vi "main_V2 _1.vi"() -> ()   [LabVIEW 2019]
doc: "This VI takes input from HMI (Nextion 7inch enhanced version) DIOs, emergency button (used as interlocking) and mode (Auto/manual) button from hardware. After getting inputs it will operate the Jacks either manual or in auto mode."
uses:
  <vilib>/myRIO/Instrument Drivers/Onboard IO/DIO/typedefs/DIO Reference.ctl
  <vilib>/myRIO/Common/Instrument Driver Framework/Utilities/typedefs/myRIO Generic Hardware Reference.ctl
  <vilib>/myRIO/Common/Instrument Driver Framework/Utilities/typedefs/Hardware Version Enum.ctl
  <vilib>/myRIO/Common/Instrument Driver Framework/Utilities/typedefs/myRIO v1.0 Reference.ctl
  <vilib>/myRIO/Common/Instrument Driver Framework/Utilities/typedefs/Generic FPGA Reference.ctl
  <vilib>/myRIO/Common/Instrument Driver Framework/myRIO v1.0/DIO/typedefs/DIO Channels List.ctl
  <vilib>/myRIO/Common/Instrument Driver Framework/myRIO v1.0/DIO/typedefs/DIO Channels Enum.ctl
  <vilib>/userDefined/High Color/nirio_resource_hc.ctl
  <vilib>/myRIO/Common/Instrument Driver Framework/Utilities/vis/Is FPGA Ref Available.vi
  <vilib>/myRIO/Common/Instrument Driver Framework/myRIO v1.0/DIO/vis/myRIO v1.1 Open DIO.vi
  <vilib>/myRIO/Instrument Drivers/Onboard IO/DIO/vis/Read.vi
  <vilib>/myRIO/Instrument Drivers/Onboard IO/DIO/vis/Write.vi
  <vilib>/myRIO/Common/Instrument Driver Framework/Utilities/vis/Validate Channels.vi
  <vilib>/myRIO/Common/Instrument Driver Framework/myRIO v1.0/DIO/vis/myRIO v1.0 Reserve DIO.vi
  <vilib>/myRIO/Common/Instrument Driver Framework/myRIO v1.0/Resource Manager/vis/myRIO v1.0 Reserve Channel List.vi
  <vilib>/myRIO/Common/Instrument Driver Framework/myRIO v1.0/DIO/vis/myRIO v1.0 Build MUX Configuration DIO.vi
  <vilib>/myRIO/Common/Instrument Driver Framework/myRIO v1.0/Resource Manager/vis/myRIO v1.0 Reserve Channel.vi
  <vilib>/myRIO/Common/Instrument Driver Framework/myRIO v1.0/Resource Manager/vis/myRIO v1.0 Unreserve Channel.vi
  <vilib>/myRIO/Common/Instrument Driver Framework/myRIO v1.0/Resource Manager/vis/myRIO v1.0 Create Configuration List.vi
  <vilib>/myRIO/Common/Instrument Driver Framework/myRIO v1.0/Resource Manager/vis/myRIO v1.0 Build Mutex Name.vi
  <vilib>/Utility/VariantDataType/GetNumericInfo.vi
  <vilib>/Utility/error.llb/Error Cluster From Error Code.vi
  <vilib>/myRIO/Common/Instrument Driver Framework/myRIO v1.0/myRIO v1.1 Open.vi
  <vilib>/myRIO/Common/Instrument Driver Framework/Utilities/vis/IO Manager.vi
  <vilib>/myRIO/Common/Instrument Driver Framework/Utilities/vis/Configuration Manager.vi
  <vilib>/myRIO/Common/Instrument Driver Framework/myRIO v1.0/Resource Manager/vis/myRIO v1.0 Configure IO.vi
  <vilib>/myRIO/Common/Instrument Driver Framework/myRIO v1.0/myRIO v1.0 Close.vi
  <vilib>/myRIO/Common/Instrument Driver Framework/myRIO v1.0/DIO/vis/myRIO v1.0 Read DIO.vi
  <vilib>/myRIO/Common/Instrument Driver Framework/myRIO v1.0/DIO/vis/myRIO v1.0 Write DIO.vi
  <vilib>/myRIO/Express VI/Onboard IO/DI/DI Express VI.xnode
  <vilib>/myRIO/Instrument Drivers/Onboard IO/DIO/vis/myRIO DIO Open.xnode
  <vilib>/myRIO/Express VI/Onboard IO/DO/DO Express VI.xnode
  <vilib>/myRIO/Instrument Drivers/Onboard IO/DIO/DIO.lvlib
panel:
  out "timerst":i32
  in  "Reset":bool
  out "Elapsed Time (s)":dbl format="%#_2g"
  out "levell check":i32
  out "1":bool
  out "X Axis":dbl
  out "Y Axis":dbl
  out "8":bool
  out "7":bool
  out "4":bool
  out "3":bool
  out "6":bool
  out "5":bool
  out "2":bool
  out "Numeric":i32
  out "Numeric 2":i32
  out "AutoLevel":bool
  out "WithDrawAll":bool
  out "Emergency stop":bool
  out "z":i16
  out "Temp":dbl
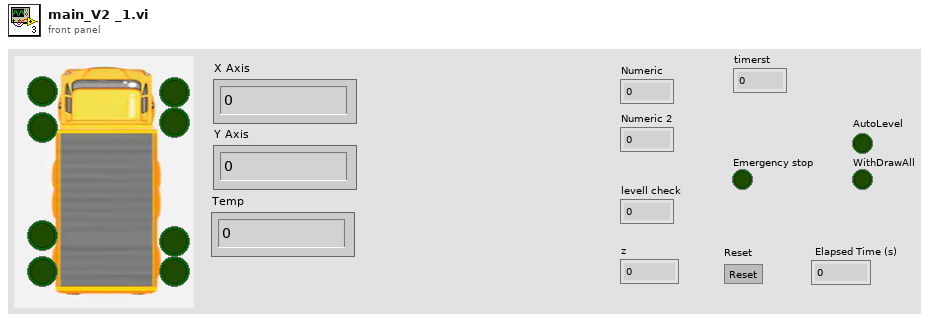
[diagram p1: front panel]
types:
  T1 = typedef "DIO.lvlib/DIO Reference.ctl" = cluster{"myRIO Reference":T2, "DIO Channels List":T6}
  T2 = typedef "myRIO Generic Hardware Reference.ctl" = cluster{"myRIO Model":T3, "myRIO Hardware Reference":T4}
  T3 = typedef "Hardware Version Enum.ctl" = enum16{"Unknown", "myRIO-1900", "myRIO-1950", "roboRIO", "NI ELVIS RIO CM", "ELVIS III"}
  T4 = typedef "myRIO v1.0 Reference.ctl" = cluster{"Generic FPGA Reference":T5, "Allow multiple opens":bool}
  T5 = typedef "Generic FPGA Reference.ctl" = refnum<k20>
  T6 = typedef "DIO Channels List.ctl" = T7[]
  T7 = typedef "DIO Channels Enum.ctl" = enum16{"Not Connected", "C/DIO0", "C/DIO1", "C/DIO2", "C/DIO3", "C/DIO4", "C/DIO5", "C/DIO6", "C/DIO7", "A/DIO0", "A/DIO1", "A/DIO2", "A/DIO3", "A/DIO4", "A/DIO5", "A/DIO6", "A/DIO7", "A/DIO8", "A/DIO9", "A/DIO10", "A/DIO11", "A/DIO12", "A/DIO13", "A/DIO14", "A/DIO15", "A/DIO16", "A/DIO17", "A/DIO18", "A/DIO19", "B/DIO0", "B/DIO1", "B/DIO2", "B/DIO3", "B/DIO4", "B/DIO5", "B/DIO6", "B/DIO7", "B/DIO8", "B/DIO9", "B/DIO10", "B/DIO11", "B/DIO12", "B/DIO13", "B/DIO14", "B/DIO15", "B/DIO16", "B/DIO17", "B/DIO18", "B/DIO19", "LED0", "LED1", "LED2", "LED3", "Button0", "DIO/DIO0", "DIO/DIO1", "DIO/DIO2", "DIO/DIO3", "DIO/DIO4", "DIO/DIO5", "DIO/DIO6", "DIO/DIO7", "DIO/DIO8", "DIO/DIO9", "SPI/CS0", "SPI/CS1", "SPI/CS2", "SPI/CS3", "LED RADIO (Green)", "LED RADIO (Red)", "LED COMM (Green)", "LED COMM (Red)", "LED MODE (Green)", "LED MODE (Red)"}
  T8 = typedef "nirio_resource_hc.ctl" = tag
  T9 = cluster{"Boolean array[0]":bool, "Boolean array[1]":bool, "Boolean array[2]":bool, "Boolean array[3]":bool, "Boolean array[4]":bool, "Boolean array[5]":bool, "Boolean array[6]":bool, "Boolean array[7]":bool}
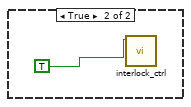
[diagram p3: hidden frame]
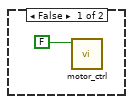
[diagram p6: hidden frame]
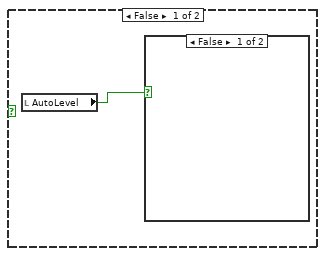
[diagram p7: hidden frame]
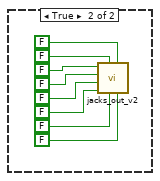
[diagram p8: hidden frame]
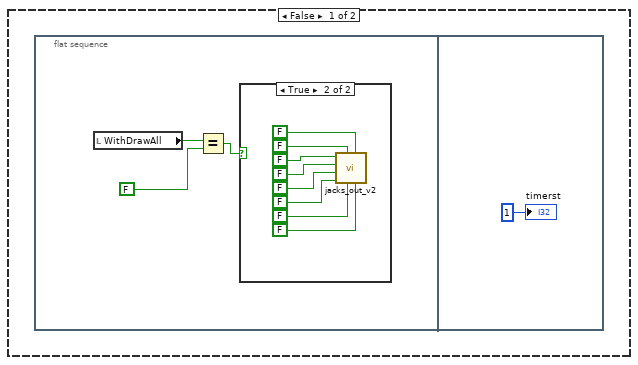
[diagram p9: hidden frame]
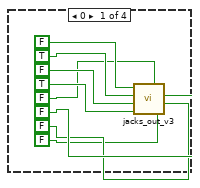
[diagram p11: hidden frame]
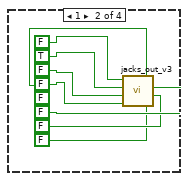
[diagram p12: hidden frame]
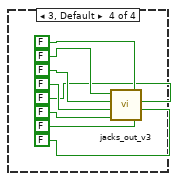
[diagram p13: hidden frame]
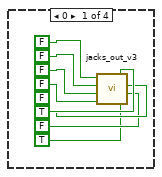
[diagram p14: hidden frame]
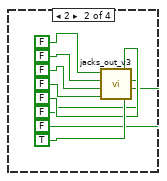
[diagram p15: hidden frame]
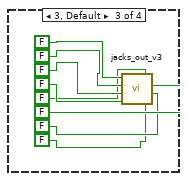
[diagram p16: hidden frame]
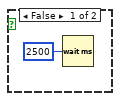
[diagram p19: hidden frame]
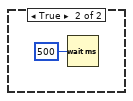
[diagram p20: hidden frame]
diagram:
  n1 = while {
    shift-right: [w16] -> _
    shift-left: 0 -> [w17]
    shift-right: [w7] -> _
    shift-left: 0 -> [w9]
    i -> [w15]
    stop <- FALSE ("stop") stop-if-true
    n2 = flat-sequence {
      tunnel: w17 -> [w21]
      tunnel: [w21] -> w14
      tunnel: [w19] -> w11
      tunnel: [w20] -> w10
      tunnel: w9 -> [w20]
      tunnel: w14 -> [w61]
      tunnel: [w60] -> w6
      tunnel: w11 -> [w59]
      tunnel: w10 -> [w58]
      tunnel: [w57] -> w5
      tunnel: w6 -> [w823]
      tunnel: [w823] -> w13
      tunnel: [w819] -> w8
      tunnel: w5 -> [w819]
      tunnel: w13 -> [w835]
      tunnel: w8 -> [w831]
      tunnel: [w835] -> w4
      tunnel: [w831] -> w3
      tunnel: [w849] -> w7
      tunnel: [w850] -> w16
      tunnel: w4 -> [w850]
      tunnel: w3 -> [w849]
      frame #0 {
        # "True for Manual and False for Auto"
        n3 = xnode "Button_inputs"() -> ("MANUAL/SFTWRE (A/DIO9 (Pin 29))"=w18:bool)  [unwired: 1 in, 1 out]
        n4 = Not(x=w18) -> (.not. x?=w19:bool)
        "Emergency stop" <- w19
      }
      frame #1 {
        # "Emergency stop case"
        n5 = case shown="True" w59 {
          tunnel: w61 -> [_ w148]
          tunnel: [0 w150] -> w60
          tunnel: w58 -> [_ w146]
          tunnel: [0 w145] -> w57
          frame False {
            n6 = flat-sequence {
              frame #0 {
                n7 = xnode "Digital output (1 sample) 4"("contactor (A/DIO3 (Pin 17))"=FALSE) -> ()  [unwired: 1 in, 1 out]
              }
              frame #1 {
                n8 = xnode "Interlock"("interlock_relay (A/DIO4 (Pin 19))"=FALSE ("interlock_relay (B/DIO8 (Pin 27))")) -> ()  [unwired: 1 in, 1 out]
              }
              frame #2 {
                n9 = call "jacks_out_v2.vi"("J4dn"=FALSE ("R6 (B/DIO13 (Pin 26))"), "J1up"=FALSE ("R3 (B/DIO2 (Pin 15))"), "J4up"=FALSE ("R5 (B/DIO4 (Pin 19))"), "J1dn"=FALSE ("R2 (B/DIO1 (Pin 13))"), "J3dn"=FALSE ("R4 (B/DIO3 (Pin 17))"), "J3up"=FALSE ("R7 (B/DIO14 (Pin 32))"), "J2dn"=FALSE ("R8 (B/DIO15 (Pin 34))"), "J2up"=FALSE ("R1 (B/DIO0 (Pin 11))")) -> ()  [unwired: 4 in]
              }
              frame #3 {
                n10 = local write "levell check"(0 ("levell check")) -> ()
              }
            }
          }
          frame True {
            n11 = flat-sequence {
              tunnel: [w154] -> w149
              tunnel: w148 -> [w154]
              tunnel: [w152] -> w147
              tunnel: w146 -> [w152]
              tunnel: [w161] -> w150
              tunnel: w149 -> [w160]
              tunnel: w147 -> [w159]
              tunnel: [w158] -> w145
              frame #0 {
                n12 = call "interlock_ctrl.vi"("Interlock"=TRUE ("interlock_relay (B/DIO8 (Pin 27))")) -> ()  [unwired: 7 in]
                n13 = Wait (ms)(milliseconds to wait=u32 50) -> ()  [unwired: 1 out]
              }
              frame #1 {
                # "Manual/Auto case"
                n14 = call "Nextion_PageRead.vi"() -> ("pageNo"=w157:u8)  [unwired: 10 in, 1 out]
                n15 = Equal?(x=w157, y=u8 1) -> (x = y?=w155:bool)
                n16 = case "Auto/Manual Case" shown="False" w155 {
                  tunnel: [w164 0] -> w161
                  tunnel: w160 -> [w162 _]
                  tunnel: w159 -> [_ w507]
                  tunnel: [0 w506] -> w158
                  frame False {
                    # "cccvv"
                    n17 = flat-sequence {
                      tunnel: w162 -> [w167]
                      frame #0 {
                        n18 = Equal?(x=w167, y=0) -> (x = y?=w165:bool)
                        n19 = case shown="True" w165 {
                          frame False {
                          }
                          frame True {
                            n20 = Wait (ms)(milliseconds to wait=u32 100) -> ()  [unwired: 1 out]
                            n21 = call "Nextion_Write.vi"("string"="page page0") -> ()  [unwired: 10 in, 1 out]
                            n22 = call "jacks_out_v3.vi"("J4 DOWN"=FALSE ("R6 (B/DIO13 (Pin 26))"), "J4 UP"=FALSE ("R5 (B/DIO4 (Pin 19))"), "J3 DOWN"=FALSE ("R4 (B/DIO3 (Pin 17))"), "J3 UP"=FALSE ("R7 (B/DIO14 (Pin 32))"), "J2 DOWN"=FALSE ("R8 (B/DIO15 (Pin 34))"), "J2 UP"=FALSE ("R1 (B/DIO0 (Pin 11))"), "J1 DOWN"=FALSE ("R2 (B/DIO1 (Pin 13))"), "J1 UP"=FALSE ("R3 (B/DIO2 (Pin 15))")) -> ()
                            "levell check" <- 0
                          }
                        }
                      }
                      frame #1 {
                        n23 = flat-sequence {
                          frame #0 {
                            n24 = call "Nextion_buttonRead.vi"("string"="get bt0.val") -> ("Bt_val"=w187:u8, "ref"=w186:u8)  [unwired: 8 in, 1 out]
                            n25 = Wait (ms)(milliseconds to wait=u32 50) -> ()  [unwired: 1 out]
                            n26 = Equal?(x=w187, y=u8 1) -> (x = y?=w185:bool)
                            n27 = Equal?(x=u8 113, y=w186) -> (x = y?=w184:bool)
                            n28 = And(x=w184, y=w185) -> (x .and. y?=→"AutoLevel":bool)
                          }
                          frame #1 {
                            n29 = call "Nextion_buttonRead.vi"("string"="get bt1.val") -> ("Bt_val"=w190:u8, "ref"=w191:u8)  [unwired: 8 in, 1 out]
                            n30 = Wait (ms)(milliseconds to wait=u32 50) -> ()  [unwired: 1 out]
                            n31 = Equal?(x=u8 113, y=w191) -> (x = y?=w193:bool)
                            n32 = Equal?(x=w190, y=u8 1) -> (x = y?=w192:bool)
                            n33 = And(x=w193, y=w192) -> (x .and. y?=→"WithDrawAll":bool)
                          }
                          frame #2 {
                            n34 = local read "WithDrawAll"() -> (w198:bool)
                            n35 = local read "AutoLevel"() -> (w199:bool)
                            n36 = Or(x=w199, y=w198) -> (x .or. y?=w197:bool)
                            n37 = case shown="True" w197 {
                              frame False {
                                n38 = call "motor_ctrl.vi"("Motor"=FALSE ("contactor (A/DIO3 (Pin 17))")) -> ()  [unwired: 7 in]
                              }
                              frame True {
                                n39 = call "motor_ctrl.vi"("Motor"=TRUE ("contactor (A/DIO3 (Pin 17))")) -> ()  [unwired: 7 in]
                              }
                            }
                          }
                          frame #3 {
                            n40 = local read "WithDrawAll"() -> (w203:bool)
                            n41 = case shown="True" w203 {
                              frame False {
                                n42 = local read "AutoLevel"() -> (w204:bool)
                                n43 = case shown="False" w204 {
                                frame False {
                                }
                                frame True {
                                n44 = call "jacks_out_v2.vi"("J4dn"=FALSE ("R6 (B/DIO13 (Pin 26))"), "J1up"=FALSE ("R3 (B/DIO2 (Pin 15))"), "J4up"=FALSE ("R5 (B/DIO4 (Pin 19))"), "J1dn"=FALSE ("R2 (B/DIO1 (Pin 13))"), "J3dn"=FALSE ("R4 (B/DIO3 (Pin 17))"), "J3up"=FALSE ("R7 (B/DIO14 (Pin 32))"), "J2dn"=FALSE ("R8 (B/DIO15 (Pin 34))"), "J2up"=FALSE ("R1 (B/DIO0 (Pin 11))")) -> ()  [unwired: 4 in]
                                }
                                }
                              }
                              frame True {
                                n45 = local write "levell check"(0 ("levell check")) -> ()
                                n46 = call "jacks_out_v3.vi"("J4 DOWN"=FALSE ("R6 (B/DIO13 (Pin 26))"), "J4 UP"=TRUE ("R5 (B/DIO4 (Pin 19))"), "J3 DOWN"=FALSE ("R4 (B/DIO3 (Pin 17))"), "J3 UP"=TRUE ("R7 (B/DIO14 (Pin 32))"), "J2 DOWN"=FALSE ("R8 (B/DIO15 (Pin 34))"), "J2 UP"=TRUE ("R1 (B/DIO0 (Pin 11))"), "J1 DOWN"=FALSE ("R2 (B/DIO1 (Pin 13))"), "J1 UP"=TRUE ("R3 (B/DIO2 (Pin 15))")) -> ()
                              }
                            }
                            n47 = Wait (ms)(milliseconds to wait=u32 50) -> ()  [unwired: 1 out]
                          }
                          frame #4 {
                          }
                          frame #5 {
                            n48 = local read "AutoLevel"() -> (w222:bool)
                            n49 = case shown="True" w222 {
                              frame False {
                                n50 = flat-sequence {
                                frame #0 {
                                n51 = local read "WithDrawAll"() -> (w224:bool)
                                n52 = Equal?(x=w224, y=FALSE) -> (x = y?=w225:bool)
                                n53 = case shown="True" w225 {
                                frame False {
                                }
                                frame True {
                                n54 = call "jacks_out_v2.vi"("J4dn"=FALSE ("R6 (B/DIO13 (Pin 26))"), "J1up"=FALSE ("R3 (B/DIO2 (Pin 15))"), "J4up"=FALSE ("R5 (B/DIO4 (Pin 19))"), "J1dn"=FALSE ("R2 (B/DIO1 (Pin 13))"), "J3dn"=FALSE ("R4 (B/DIO3 (Pin 17))"), "J3up"=FALSE ("R7 (B/DIO14 (Pin 32))"), "J2dn"=FALSE ("R8 (B/DIO15 (Pin 34))"), "J2up"=FALSE ("R1 (B/DIO0 (Pin 11))")) -> ()  [unwired: 4 in]
                                }
                                }
                                }
                                frame #1 {
                                "timerst" <- 1
                                }
                                }
                              }
                              frame True {
                                n55 = flat-sequence {
                                frame #0 {
                                n56 = local read "timerst"() -> (w240:i32)
                                n57 = Equal?(x=w240, y=1) -> (x = y?=w235:bool)
                                n58 = Select(t=TRUE ("Reset"), s=w235, f=FALSE ("Reset")) -> (s? t:f=w238:bool)
                                n59 = local write "Reset"(w238) -> ()
                                }
                                frame #1 {
                                n60 = flat-sequence {
                                tunnel: [w242] -> w241
                                tunnel: w241 -> [w244]
                                frame #0 {
                                n61 = call "Elapsed Time"("Reset"="Reset") -> ("Elapsed Time (s)"=w242:dbl)  [unwired: 11 in, 7 out]
                                "Elapsed Time (s)" <- w242
                                }
                                frame #1 {
                                n62 = Multiply(x=w244, y=10.0) -> (x*y=w246:dbl)
                                n63 = To Word Integer(number=w246) -> (16bit integer=w245:i16)
                                n64 = Format Into String(initial string="x2.val=", w245) -> (resulting string=w248:string)  [unwired: 2 in, 1 out]
                                n65 = call "Nextion_Write.vi"("string"=w248) -> ()  [unwired: 10 in, 1 out]
                                }
                                frame #2 {
                                n66 = Format Into String(initial string="t4.bco=", 0 ("input 1")) -> (resulting string=w251:string)  [unwired: 2 in, 1 out]
                                n67 = call "Nextion_Write.vi"("string"=w251) -> ()  [unwired: 10 in, 1 out]
                                }
                                frame #3 {
                                n68 = local write "timerst"(0 ("timerst")) -> ()
                                }
                                }
                                }
                                frame #2 {
                                n69 = local write "levell check"(0 ("levell check")) -> ()
                                }
                                frame #3 {
                                n70 = while {
                                stop <- w280 stop-if-true
                                # "Opening the Jacks one by one till ground touch then start Auto leveling."
                                n71 = call "Jacks_SensorOut.vi"() -> ("J2Sensor"=w256:bool, "J1Sensor"=w257:bool)  [unwired: 8 in, 2 out]
                                n72 = Build Array(w257, w256) -> (w272:bool[])
                                n73 = Boolean To (0,1)(Boolean=w257) -> (0, 1=w263:i16)
                                n74 = Boolean Array To Number(Boolean array=w272) -> (number=w270:u32)
                                n75 = Boolean To (0,1)(Boolean=w256) -> (0, 1=w262:i16)
                                n76 = Format Into String(initial string="b11.val=", w263) -> (resulting string=w264:string)  [unwired: 2 in, 1 out]
                                n77 = Format Into String(initial string="b9.val=", w262) -> (resulting string=w261:string)  [unwired: 2 in, 1 out]
                                n78 = call "Nextion_Write.vi"("string"=w264) -> ("error out"=w259:errorcluster)  [unwired: 10 in]
                                n79 = call "Nextion_Write.vi"("error in (no error)"=w259, "string"=w261) -> ("error out"=w258:errorcluster)  [unwired: 9 in]
                                n80 = In Range and Coerce(upper limit=u32 3 ("x"), x=w270, lower limit=u32 0) -> (In Range?=w267:bool)  [unwired: 1 out]
                                n81 = Not(x=w267) -> (.not. x?=w266:bool)
                                n82 = case shown="2" w270 {
                                frame 0 {
                                n83 = call "jacks_out_v3.vi"("J4 DOWN"=FALSE ("R6 (B/DIO13 (Pin 26))"), "J4 UP"=FALSE ("R5 (B/DIO4 (Pin 19))"), "J3 DOWN"=FALSE ("R4 (B/DIO3 (Pin 17))"), "J3 UP"=FALSE ("R7 (B/DIO14 (Pin 32))"), "J2 DOWN"=TRUE ("R8 (B/DIO15 (Pin 34))"), "J2 UP"=FALSE ("R1 (B/DIO0 (Pin 11))"), "J1 DOWN"=TRUE ("R2 (B/DIO1 (Pin 13))"), "J1 UP"=FALSE ("R3 (B/DIO2 (Pin 15))")) -> ()
                                }
                                frame 1 {
                                n84 = call "jacks_out_v3.vi"("J4 DOWN"=FALSE ("R6 (B/DIO13 (Pin 26))"), "J4 UP"=FALSE ("R5 (B/DIO4 (Pin 19))"), "J3 DOWN"=FALSE ("R4 (B/DIO3 (Pin 17))"), "J3 UP"=FALSE ("R7 (B/DIO14 (Pin 32))"), "J2 DOWN"=FALSE ("R8 (B/DIO15 (Pin 34))"), "J2 UP"=FALSE ("R1 (B/DIO0 (Pin 11))"), "J1 DOWN"=TRUE ("R2 (B/DIO1 (Pin 13))"), "J1 UP"=FALSE ("R3 (B/DIO2 (Pin 15))")) -> ()
                                }
                                frame 2 {
                                n85 = call "jacks_out_v3.vi"("J4 DOWN"=FALSE ("R6 (B/DIO13 (Pin 26))"), "J4 UP"=FALSE ("R5 (B/DIO4 (Pin 19))"), "J3 DOWN"=FALSE ("R4 (B/DIO3 (Pin 17))"), "J3 UP"=FALSE ("R7 (B/DIO14 (Pin 32))"), "J2 DOWN"=TRUE ("R8 (B/DIO15 (Pin 34))"), "J2 UP"=FALSE ("R1 (B/DIO0 (Pin 11))"), "J1 DOWN"=FALSE ("R2 (B/DIO1 (Pin 13))"), "J1 UP"=FALSE ("R3 (B/DIO2 (Pin 15))")) -> ()
                                }
                                frame 3, Default {
                                n86 = call "jacks_out_v3.vi"("J4 DOWN"=FALSE ("R5 (B/DIO4 (Pin 19))"), "J4 UP"=FALSE ("R6 (B/DIO13 (Pin 26))"), "J3 DOWN"=FALSE ("R7 (B/DIO14 (Pin 32))"), "J3 UP"=FALSE ("R3 (B/DIO2 (Pin 15))"), "J2 DOWN"=FALSE ("R4 (B/DIO3 (Pin 17))"), "J2 UP"=FALSE ("R8 (B/DIO15 (Pin 34))"), "J1 DOWN"=FALSE ("R1 (B/DIO0 (Pin 11))"), "J1 UP"=FALSE ("R2 (B/DIO1 (Pin 13))")) -> ()
                                }
                                }
                                n87 = xnode "Emrgency"() -> ("Emergency stop (B/DIO8 (Pin 27))"=w255:bool)  [unwired: 1 in, 1 out]
                                n88 = call "Nextion_buttonRead.vi"("error in (no error)"=w258, "string"="get bt0.val") -> ("Bt_val"=w279:u8, "ref"=w278:u8)  [unwired: 7 in, 1 out]
                                n89 = Equal?(x=w279, y=u8 0) -> (x = y?=w277:bool)
                                n90 = Equal?(x=u8 113, y=w278) -> (x = y?=w276:bool)
                                n91 = And(x=w276, y=w277) -> (x .and. y?=w271:bool)
                                n92 = Compound Arithmetic op=OR(w266, w271, w255) -> (w280:bool)
                                }
                                }
                                frame #4 {
                                n93 = while {
                                stop <- w366 stop-if-true
                                n94 = call "Jacks_SensorOut.vi"() -> ("J4Sensor"=w349:bool, "J3Sensor"=w350:bool)  [unwired: 8 in, 2 out]
                                n95 = Build Array(w350, w349) -> (w359:bool[])
                                n96 = Boolean To (0,1)(Boolean=w349) -> (0, 1=w355:i16)
                                n97 = Boolean Array To Number(Boolean array=w359) -> (number=w361:u32)
                                n98 = Boolean To (0,1)(Boolean=w350) -> (0, 1=w357:i16)
                                n99 = Format Into String(initial string="b10.val=", w355) -> (resulting string=w356:string)  [unwired: 2 in, 1 out]
                                n100 = call "Nextion_Write.vi"("string"=w356) -> ("error out"=w352:errorcluster)  [unwired: 10 in]
                                n101 = Format Into String(initial string="b12.val=", w357) -> (resulting string=w358:string)  [unwired: 2 in, 1 out]
                                n102 = call "Nextion_Write.vi"("error in (no error)"=w352, "string"=w358) -> ("error out"=w351:errorcluster)  [unwired: 9 in]
                                n103 = In Range and Coerce(upper limit=u32 3 ("x"), x=w361, lower limit=u32 0) -> (In Range?=w362:bool)  [unwired: 1 out]
                                n104 = case shown="1" w361 {
                                frame 0 {
                                n105 = call "jacks_out_v3.vi"("J4 DOWN"=TRUE ("R6 (B/DIO13 (Pin 26))"), "J4 UP"=FALSE ("R5 (B/DIO4 (Pin 19))"), "J3 DOWN"=TRUE ("R4 (B/DIO3 (Pin 17))"), "J3 UP"=FALSE ("R7 (B/DIO14 (Pin 32))"), "J2 DOWN"=FALSE ("R8 (B/DIO15 (Pin 34))"), "J2 UP"=FALSE ("R1 (B/DIO0 (Pin 11))"), "J1 DOWN"=FALSE ("R2 (B/DIO1 (Pin 13))"), "J1 UP"=FALSE ("R3 (B/DIO2 (Pin 15))")) -> ()
                                }
                                frame 2 {
                                n106 = call "jacks_out_v3.vi"("J4 DOWN"=TRUE ("R6 (B/DIO13 (Pin 26))"), "J4 UP"=FALSE ("R5 (B/DIO4 (Pin 19))"), "J3 DOWN"=FALSE ("R4 (B/DIO3 (Pin 17))"), "J3 UP"=FALSE ("R7 (B/DIO14 (Pin 32))"), "J2 DOWN"=FALSE ("R8 (B/DIO15 (Pin 34))"), "J2 UP"=FALSE ("R1 (B/DIO0 (Pin 11))"), "J1 DOWN"=FALSE ("R2 (B/DIO1 (Pin 13))"), "J1 UP"=FALSE ("R3 (B/DIO2 (Pin 15))")) -> ()
                                }
                                frame 3, Default {
                                n107 = call "jacks_out_v3.vi"("J4 DOWN"=FALSE ("R6 (B/DIO13 (Pin 26))"), "J4 UP"=FALSE ("R5 (B/DIO4 (Pin 19))"), "J3 DOWN"=FALSE ("R4 (B/DIO3 (Pin 17))"), "J3 UP"=FALSE ("R7 (B/DIO14 (Pin 32))"), "J2 DOWN"=FALSE ("R8 (B/DIO15 (Pin 34))"), "J2 UP"=FALSE ("R1 (B/DIO0 (Pin 11))"), "J1 DOWN"=FALSE ("R2 (B/DIO1 (Pin 13))"), "J1 UP"=FALSE ("R3 (B/DIO2 (Pin 15))")) -> ()
                                }
                                frame 1 {
                                n108 = call "jacks_out_v3.vi"("J4 DOWN"=FALSE ("R6 (B/DIO13 (Pin 26))"), "J4 UP"=FALSE ("R5 (B/DIO4 (Pin 19))"), "J3 DOWN"=TRUE ("R4 (B/DIO3 (Pin 17))"), "J3 UP"=FALSE ("R7 (B/DIO14 (Pin 32))"), "J2 DOWN"=FALSE ("R8 (B/DIO15 (Pin 34))"), "J2 UP"=FALSE ("R1 (B/DIO0 (Pin 11))"), "J1 DOWN"=FALSE ("R2 (B/DIO1 (Pin 13))"), "J1 UP"=FALSE ("R3 (B/DIO2 (Pin 15))")) -> ()
                                }
                                }
                                n109 = Not(x=w362) -> (.not. x?=w360:bool)
                                n110 = call "Nextion_buttonRead.vi"("error in (no error)"=w351, "string"="get bt0.val") -> ("Bt_val"=w373:u8, "ref"=w372:u8)  [unwired: 7 in, 1 out]
                                n111 = xnode "Emrgency"() -> ("Emergency stop (B/DIO8 (Pin 27))"=w348:bool)  [unwired: 1 in, 1 out]
                                n112 = Equal?(x=w373, y=u8 0) -> (x = y?=w371:bool)
                                n113 = Equal?(x=u8 113, y=w372) -> (x = y?=w370:bool)
                                n114 = And(x=w370, y=w371) -> (x .and. y?=w365:bool)
                                n115 = Compound Arithmetic op=OR(w360, w365, w348) -> (w366:bool)
                                }
                                }
                                frame #5 {
                                n116 = call "jacks_out_v3.vi"("J4 DOWN"=FALSE ("R6 (B/DIO13 (Pin 26))"), "J4 UP"=FALSE ("R5 (B/DIO4 (Pin 19))"), "J3 DOWN"=FALSE ("R4 (B/DIO3 (Pin 17))"), "J3 UP"=FALSE ("R7 (B/DIO14 (Pin 32))"), "J2 DOWN"=FALSE ("R8 (B/DIO15 (Pin 34))"), "J2 UP"=FALSE ("R1 (B/DIO0 (Pin 11))"), "J1 DOWN"=FALSE ("R2 (B/DIO1 (Pin 13))"), "J1 UP"=FALSE ("R3 (B/DIO2 (Pin 15))")) -> ()
                                }
                                frame #6 {
                                n117 = local read "Temp"() -> (w451:dbl)
                                n118 = Not Equal?(x=w451, y=0.0) -> (x != y?=w449:bool)
                                n119 = case shown="True" w449 {
                                frame False {
                                }
                                frame True {
                                n120 = flat-sequence {
                                frame #0 {
                                n121 = local read "X Axis"() -> (w461:dbl)
                                n122 = local read "Y Axis"() -> (w466:dbl)
                                n123 = call "Truck_inclination_quadrantFind.vi"("y"=w466, "x"=w461) -> ("z"=w460:i16)  [unwired: 9 in]
                                "z" <- w460
                                n124 = Number To Boolean Array(number=w460) -> (Boolean array=w465:bool[])
                                n125 = Reshape Array(w465, 8 ("dimension size")) -> (w463:bool[])
                                n126 = Array To Cluster(array=w463) -> (cluster=w462:T9)
                                n127 = Unbundle(w462) -> ("Boolean array[0]"=w459:bool, "Boolean array[1]"=w458:bool, "Boolean array[2]"=w457:bool, "Boolean array[3]"=w456:bool, "Boolean array[4]"=w455:bool, "Boolean array[5]"=w454:bool, "Boolean array[6]"=w453:bool, "Boolean array[7]"=w452:bool)
                                n128 = call "jacks_out_v3.vi"("J4 DOWN"=w452, "J4 UP"=w453, "J3 DOWN"=w454, "J3 UP"=w455, "J2 DOWN"=w456, "J2 UP"=w457, "J1 DOWN"=w458, "J1 UP"=w459) -> ()
                                }
                                frame #1 {
                                n129 = local read "z"() -> (w468:i16)
                                n130 = Equal?(x=w468, y=i16 0) -> (x = y?=w469:bool)
                                n131 = case shown="True" w469 {
                                frame False {
                                }
                                frame True {
                                n132 = flat-sequence {
                                frame #0 {
                                n133 = local write "levell check"(1 ("levell check")) -> ()
                                n134 = call "Nextion_Write.vi"("string"="bt0.val=0") -> ()  [unwired: 10 in, 1 out]
                                }
                                frame #1 {
                                n135 = local read "Elapsed Time (s)"() -> (w472:dbl)
                                n136 = Multiply(x=w472, y=10.0) -> (x*y=w474:dbl)
                                n137 = To Word Integer(number=w474) -> (16bit integer=w473:i16)
                                n138 = Format Into String(initial string="x2.val=", w473) -> (resulting string=w476:string)  [unwired: 2 in, 1 out]
                                n139 = call "Nextion_Write.vi"("string"=w476) -> ()  [unwired: 10 in, 1 out]
                                }
                                frame #2 {
                                n140 = Format Into String(initial string="t4.bco=", 0 ("input 1")) -> (resulting string=w479:string)  [unwired: 2 in, 1 out]
                                n141 = call "Nextion_Write.vi"("string"=w479) -> ()  [unwired: 10 in, 1 out]
                                }
                                }
                                }
                                }
                                }
                                frame #2 {
                                n142 = local read "X Axis"() -> (w487:dbl)
                                n143 = local read "Y Axis"() -> (w483:dbl)
                                n144 = call "auto_jackTime_find.vi"("UL-X"=1.0, "x"=w487, "LL-X"=-1.0, "UL-Y"=1.0, "y"=w483, "LL-Y"=-1.0) -> (17:w481:bool)  [unwired: 13 in]
                                n145 = case shown="False" w481 {
                                frame False {
                                n146 = local read "X Axis"() -> (w489:dbl)
                                n147 = local read "Y Axis"() -> (w488:dbl)
                                n148 = call "auto_jackTime_find.vi"("UL-X"=2.0, "x"=w489, "LL-X"=-2.0, "UL-Y"=2.0, "y"=w488, "LL-Y"=-2.0) -> (17:w490:bool)  [unwired: 13 in]
                                n149 = case shown="True" w490 {
                                frame False {
                                n150 = Wait (ms)(milliseconds to wait=u32 2500) -> ()  [unwired: 1 out]
                                }
                                frame True {
                                n151 = Wait (ms)(milliseconds to wait=u32 1500) -> ()  [unwired: 1 out]
                                }
                                }
                                }
                                frame True {
                                n152 = Wait (ms)(milliseconds to wait=u32 500) -> ()  [unwired: 1 out]
                                }
                                }
                                }
                                frame #3 {
                                n153 = call "jacks_out_v3.vi"("J4 DOWN"=FALSE ("R6 (B/DIO13 (Pin 26))"), "J4 UP"=FALSE ("R5 (B/DIO4 (Pin 19))"), "J3 DOWN"=FALSE ("R4 (B/DIO3 (Pin 17))"), "J3 UP"=FALSE ("R7 (B/DIO14 (Pin 32))"), "J2 DOWN"=FALSE ("R8 (B/DIO15 (Pin 34))"), "J2 UP"=FALSE ("R1 (B/DIO0 (Pin 11))"), "J1 DOWN"=FALSE ("R2 (B/DIO1 (Pin 13))"), "J1 UP"=FALSE ("R3 (B/DIO2 (Pin 15))")) -> ()
                                }
                                }
                                }
                                }
                                }
                                }
                              }
                            }
                          }
                        }
                      }
                    }
                    n154 = Increment(x=w162) -> (x+1=w164:i32)
                  }
                  frame True {
                    # "cvxcv"
                    n155 = flat-sequence {
                      tunnel: w507 -> [w510]
                      frame #0 {
                        n156 = Equal To 0?(x=w510) -> (x = 0?=w511:bool)
                        n157 = case shown="True" w511 {
                          frame False {
                          }
                          frame True {
                            n158 = call "Nextion_Write.vi"("string"="page page1") -> ()  [unwired: 10 in, 1 out]
                          }
                        }
                        n159 = Wait (ms)(milliseconds to wait=u32 50) -> ()  [unwired: 1 out]
                      }
                      frame #1 {
                        n160 = call "motor_ctrl.vi"("Motor"=TRUE ("contactor (A/DIO3 (Pin 17))")) -> ()  [unwired: 7 in]
                      }
                      frame #2 {
                        n161 = call "Nextion_buttonRead.vi"("string"="get bt10.val") -> ("Bt_val"=w521:u8, "ref"=w520:u8)  [unwired: 8 in, 1 out]
                        n162 = Equal?(x=w521, y=u8 1) -> (x = y?=w519:bool)
                        n163 = Equal?(x=u8 113, y=w520) -> (x = y?=w518:bool)
                        n164 = And(x=w518, y=w519) -> (x .and. y?=w514:bool)
                        n165 = case shown="True" w514 {
                          frame False {
                          }
                          frame True {
                            n166 = while {
                              stop <- w547 stop-if-true
                              # "Opening the Jacks one by one till ground touch then start Auto leveling."
                              n167 = call "Jacks_SensorOut.vi"() -> ("J2Sensor"=w523:bool, "J1Sensor"=w524:bool)  [unwired: 8 in, 2 out]
                              n168 = Build Array(w524, w523) -> (w533:bool[])
                              n169 = Boolean Array To Number(Boolean array=w533) -> (number=w538:u32)
                              n170 = Boolean To (0,1)(Boolean=w524) -> (0, 1=w530:i16)
                              n171 = Format Into String(initial string="b14.val=", w530) -> (resulting string=w531:string)  [unwired: 2 in, 1 out]
                              n172 = Boolean To (0,1)(Boolean=w523) -> (0, 1=w527:i16)
                              n173 = call "Nextion_Write.vi"("string"=w531) -> ("error out"=w526:errorcluster)  [unwired: 10 in]
                              n174 = Format Into String(initial string="b13.val=", w527) -> (resulting string=w528:string)  [unwired: 2 in, 1 out]
                              n175 = In Range and Coerce(upper limit=u32 3 ("x"), x=w538, lower limit=u32 0) -> (In Range?=w535:bool)  [unwired: 1 out]
                              n176 = Not(x=w535) -> (.not. x?=w534:bool)
                              n177 = call "Nextion_Write.vi"("error in (no error)"=w526, "string"=w528) -> ("error out"=w525:errorcluster)  [unwired: 9 in]
                              n178 = case shown="0" w538 {
                                frame 0 {
                                n179 = call "jacks_out_v3.vi"("J4 DOWN"=FALSE ("R6 (B/DIO13 (Pin 26))"), "J4 UP"=FALSE ("R5 (B/DIO4 (Pin 19))"), "J3 DOWN"=FALSE ("R4 (B/DIO3 (Pin 17))"), "J3 UP"=FALSE ("R7 (B/DIO14 (Pin 32))"), "J2 DOWN"=TRUE ("R8 (B/DIO15 (Pin 34))"), "J2 UP"=FALSE ("R1 (B/DIO0 (Pin 11))"), "J1 DOWN"=TRUE ("R2 (B/DIO1 (Pin 13))"), "J1 UP"=FALSE ("R3 (B/DIO2 (Pin 15))")) -> ()
                                }
                                frame 1 {
                                n180 = call "jacks_out_v3.vi"("J4 DOWN"=FALSE ("R6 (B/DIO13 (Pin 26))"), "J4 UP"=FALSE ("R5 (B/DIO4 (Pin 19))"), "J3 DOWN"=FALSE ("R4 (B/DIO3 (Pin 17))"), "J3 UP"=FALSE ("R7 (B/DIO14 (Pin 32))"), "J2 DOWN"=FALSE ("R8 (B/DIO15 (Pin 34))"), "J2 UP"=FALSE ("R1 (B/DIO0 (Pin 11))"), "J1 DOWN"=TRUE ("R2 (B/DIO1 (Pin 13))"), "J1 UP"=FALSE ("R3 (B/DIO2 (Pin 15))")) -> ()
                                }
                                frame 2 {
                                n181 = call "jacks_out_v3.vi"("J4 DOWN"=FALSE ("R6 (B/DIO13 (Pin 26))"), "J4 UP"=FALSE ("R5 (B/DIO4 (Pin 19))"), "J3 DOWN"=FALSE ("R4 (B/DIO3 (Pin 17))"), "J3 UP"=FALSE ("R7 (B/DIO14 (Pin 32))"), "J2 DOWN"=TRUE ("R8 (B/DIO15 (Pin 34))"), "J2 UP"=FALSE ("R1 (B/DIO0 (Pin 11))"), "J1 DOWN"=FALSE ("R2 (B/DIO1 (Pin 13))"), "J1 UP"=FALSE ("R3 (B/DIO2 (Pin 15))")) -> ()
                                }
                                frame 3, Default {
                                n182 = call "jacks_out_v3.vi"("J4 DOWN"=FALSE ("R6 (B/DIO13 (Pin 26))"), "J4 UP"=FALSE ("R5 (B/DIO4 (Pin 19))"), "J3 DOWN"=FALSE ("R4 (B/DIO3 (Pin 17))"), "J3 UP"=FALSE ("R7 (B/DIO14 (Pin 32))"), "J2 DOWN"=FALSE ("R8 (B/DIO15 (Pin 34))"), "J2 UP"=FALSE ("R1 (B/DIO0 (Pin 11))"), "J1 DOWN"=FALSE ("R2 (B/DIO1 (Pin 13))"), "J1 UP"=FALSE ("R3 (B/DIO2 (Pin 15))")) -> ()
                                }
                              }
                              n183 = xnode "Emrgency"() -> ("Emergency stop (B/DIO8 (Pin 27))"=w522:bool)  [unwired: 1 in, 1 out]
                              n184 = call "Nextion_buttonRead.vi"("error in (no error)"=w525, "string"="get bt10.val") -> ("Bt_val"=w546:u8, "ref"=w545:u8)  [unwired: 7 in, 1 out]
                              n185 = Equal?(x=w546, y=u8 0) -> (x = y?=w544:bool)
                              n186 = Equal?(x=u8 113, y=w545) -> (x = y?=w543:bool)
                              n187 = And(x=w543, y=w544) -> (x .and. y?=w539:bool)
                              n188 = Compound Arithmetic op=OR(w534, w539, w522) -> (w547:bool)
                            }
                          }
                        }
                      }
                      frame #3 {
                        n189 = call "Nextion_buttonRead.vi"("string"="get bt10.val") -> ("Bt_val"=w622:u8, "ref"=w621:u8)  [unwired: 8 in, 1 out]
                        n190 = Equal?(x=w622, y=u8 1) -> (x = y?=w620:bool)
                        n191 = Equal?(x=u8 113, y=w621) -> (x = y?=w619:bool)
                        n192 = And(x=w619, y=w620) -> (x .and. y?=w615:bool)
                        n193 = case shown="True" w615 {
                          frame False {
                          }
                          frame True {
                            n194 = while {
                              stop <- w641 stop-if-true
                              n195 = call "Jacks_SensorOut.vi"() -> ("J4Sensor"=w624:bool, "J3Sensor"=w625:bool)  [unwired: 8 in, 2 out]
                              n196 = Build Array(w625, w624) -> (w634:bool[])
                              n197 = Boolean To (0,1)(Boolean=w625) -> (0, 1=w631:i16)
                              n198 = Boolean Array To Number(Boolean array=w634) -> (number=w636:u32)
                              n199 = Format Into String(initial string="b16.val=", w631) -> (resulting string=w632:string)  [unwired: 2 in, 1 out]
                              n200 = Boolean To (0,1)(Boolean=w624) -> (0, 1=w628:i16)
                              n201 = call "Nextion_Write.vi"("string"=w632) -> ("error out"=w627:errorcluster)  [unwired: 10 in]
                              n202 = Format Into String(initial string="b15.val=", w628) -> (resulting string=w629:string)  [unwired: 2 in, 1 out]
                              n203 = In Range and Coerce(upper limit=u32 3 ("x"), x=w636, lower limit=u32 0) -> (In Range?=w637:bool)  [unwired: 1 out]
                              n204 = call "Nextion_Write.vi"("error in (no error)"=w627, "string"=w629) -> ("error out"=w626:errorcluster)  [unwired: 9 in]
                              n205 = Not(x=w637) -> (.not. x?=w635:bool)
                              n206 = xnode "Emrgency"() -> ("Emergency stop (B/DIO8 (Pin 27))"=w623:bool)  [unwired: 1 in, 1 out]
                              n207 = case shown="2" w636 {
                                frame 0 {
                                n208 = call "jacks_out_v3.vi"("J4 DOWN"=TRUE ("R6 (B/DIO13 (Pin 26))"), "J4 UP"=FALSE ("R5 (B/DIO4 (Pin 19))"), "J3 DOWN"=TRUE ("R4 (B/DIO3 (Pin 17))"), "J3 UP"=FALSE ("R7 (B/DIO14 (Pin 32))"), "J2 DOWN"=FALSE ("R8 (B/DIO15 (Pin 34))"), "J2 UP"=FALSE ("R1 (B/DIO0 (Pin 11))"), "J1 DOWN"=FALSE ("R2 (B/DIO1 (Pin 13))"), "J1 UP"=FALSE ("R3 (B/DIO2 (Pin 15))")) -> ()
                                }
                                frame 2 {
                                n209 = call "jacks_out_v3.vi"("J4 DOWN"=TRUE ("R6 (B/DIO13 (Pin 26))"), "J4 UP"=FALSE ("R5 (B/DIO4 (Pin 19))"), "J3 DOWN"=FALSE ("R4 (B/DIO3 (Pin 17))"), "J3 UP"=FALSE ("R7 (B/DIO14 (Pin 32))"), "J2 DOWN"=FALSE ("R8 (B/DIO15 (Pin 34))"), "J2 UP"=FALSE ("R1 (B/DIO0 (Pin 11))"), "J1 DOWN"=FALSE ("R2 (B/DIO1 (Pin 13))"), "J1 UP"=FALSE ("R3 (B/DIO2 (Pin 15))")) -> ()
                                }
                                frame 3, Default {
                                n210 = call "jacks_out_v3.vi"("J4 DOWN"=FALSE ("R6 (B/DIO13 (Pin 26))"), "J4 UP"=FALSE ("R5 (B/DIO4 (Pin 19))"), "J3 DOWN"=FALSE ("R4 (B/DIO3 (Pin 17))"), "J3 UP"=FALSE ("R7 (B/DIO14 (Pin 32))"), "J2 DOWN"=FALSE ("R8 (B/DIO15 (Pin 34))"), "J2 UP"=FALSE ("R1 (B/DIO0 (Pin 11))"), "J1 DOWN"=FALSE ("R2 (B/DIO1 (Pin 13))"), "J1 UP"=FALSE ("R3 (B/DIO2 (Pin 15))")) -> ()
                                }
                                frame 1 {
                                n211 = call "jacks_out_v3.vi"("J4 DOWN"=FALSE ("R6 (B/DIO13 (Pin 26))"), "J4 UP"=FALSE ("R5 (B/DIO4 (Pin 19))"), "J3 DOWN"=TRUE ("R4 (B/DIO3 (Pin 17))"), "J3 UP"=FALSE ("R7 (B/DIO14 (Pin 32))"), "J2 DOWN"=FALSE ("R8 (B/DIO15 (Pin 34))"), "J2 UP"=FALSE ("R1 (B/DIO0 (Pin 11))"), "J1 DOWN"=FALSE ("R2 (B/DIO1 (Pin 13))"), "J1 UP"=FALSE ("R3 (B/DIO2 (Pin 15))")) -> ()
                                }
                              }
                              n212 = call "Nextion_buttonRead.vi"("error in (no error)"=w626, "string"="get bt10.val") -> ("Bt_val"=w648:u8, "ref"=w647:u8)  [unwired: 7 in, 1 out]
                              n213 = Equal?(x=w648, y=u8 0) -> (x = y?=w646:bool)
                              n214 = Equal?(x=u8 113, y=w647) -> (x = y?=w645:bool)
                              n215 = And(x=w645, y=w646) -> (x .and. y?=w640:bool)
                              n216 = Compound Arithmetic op=OR(w635, w640, w623) -> (w641:bool)
                            }
                          }
                        }
                      }
                      frame #4 {
                        # "manual control"
                        n217 = call "Nextion_buttonRead.vi"("string"="get bt8.val") -> ("Bt_val"=w724:u8, "ref"=w723:u8)  [unwired: 8 in, 1 out]
                        n218 = Equal?(x=w724, y=u8 0) -> (x = y?=w722:bool)
                        n219 = Wait (ms)(milliseconds to wait=u32 50) -> ()  [unwired: 1 out]
                        n220 = Equal?(x=u8 113, y=w723) -> (x = y?=w721:bool)
                        n221 = And(x=w721, y=w722) -> (x .and. y?=w717:bool)
                        n222 = case shown="True" w717 {
                          frame False {
                            n223 = disable-structure shown="Disabled" {
                              frame Disabled {
                                n224 = xnode "Relay out"("R1 (B/DIO0 (Pin 11))"=TRUE, "R2 (B/DIO1 (Pin 13))"=TRUE, "R3 (B/DIO2 (Pin 15))"=TRUE, "R4 (B/DIO3 (Pin 17))"=TRUE, "R5 (B/DIO4 (Pin 19))"=TRUE, "R6 (B/DIO5 (Pin 21))"=TRUE, "R7 (B/DIO6 (Pin 23))"=TRUE, "R8 (B/DIO7 (Pin 25))"=TRUE) -> ()  [unwired: 1 in, 1 out]
                              }
                              frame Enabled {
                              }
                            }
                          }
                          frame True {
                            n225 = call "Nextion_JacksInput_UART.vi"() -> ("b7"=w776:bool, "b8"=w775:bool, "b1"=w782:bool, "b2"=w781:bool, "b3"=w780:bool, "b4"=w779:bool, "b5"=w778:bool, "b6"=w777:bool)  [unwired: 12 in]
                            "1" <- w782
                            "2" <- w781
                            "3" <- w780
                            "4" <- w779
                            "8" <- w775
                            "7" <- w776
                            "5" <- w778
                            "6" <- w777
                            n226 = call "jacks_out_v3.vi"("J4 DOWN"=w775, "J4 UP"=w776, "J3 DOWN"=w777, "J3 UP"=w778, "J2 DOWN"=w779, "J2 UP"=w780, "J1 DOWN"=w781, "J1 UP"=w782) -> ()
                          }
                        }
                      }
                      frame #5 {
                        # "withdraw all"
                        n227 = call "Nextion_buttonRead.vi"("string"="get bt8.val") -> ("Bt_val"=w791:u8, "ref"=w790:u8)  [unwired: 8 in, 1 out]
                        n228 = Wait (ms)(milliseconds to wait=u32 50) -> ()  [unwired: 1 out]
                        n229 = Equal?(x=w791, y=u8 1) -> (x = y?=w789:bool)
                        n230 = Equal?(x=u8 113, y=w790) -> (x = y?=w788:bool)
                        n231 = And(x=w788, y=w789) -> (x .and. y?=w784:bool)
                        n232 = case shown="True" w784 {
                          frame False {
                          }
                          frame True {
                            n233 = call "jacks_out_v3.vi"("J4 DOWN"=FALSE ("R6 (B/DIO13 (Pin 26))"), "J4 UP"=TRUE ("R5 (B/DIO4 (Pin 19))"), "J3 DOWN"=FALSE ("R4 (B/DIO3 (Pin 17))"), "J3 UP"=TRUE ("R7 (B/DIO14 (Pin 32))"), "J2 DOWN"=FALSE ("R8 (B/DIO15 (Pin 34))"), "J2 UP"=TRUE ("R1 (B/DIO0 (Pin 11))"), "J1 DOWN"=FALSE ("R2 (B/DIO1 (Pin 13))"), "J1 UP"=TRUE ("R3 (B/DIO2 (Pin 15))")) -> ()
                          }
                        }
                      }
                      frame #6 {
                        n234 = local write "levell check"(0 ("levell check")) -> ()
                        n235 = Wait (ms)(milliseconds to wait=u32 50) -> ()  [unwired: 1 out]
                      }
                      frame #7 {
                        n236 = call "Nextion_buttonRead.vi"("string"="get bt8.val") -> ("Bt_val"=w809:u8, "ref"=w808:u8)  [unwired: 8 in, 1 out]
                        n237 = Equal?(x=w809, y=u8 0) -> (x = y?=w807:bool)
                        n238 = Equal?(x=u8 113, y=w808) -> (x = y?=w806:bool)
                        n239 = And(x=w806, y=w807) -> (x .and. y?=w802:bool)
                        n240 = case shown="True" w802 {
                          frame False {
                          }
                          frame True {
                            n241 = call "jacks_out_v3.vi"("J4 DOWN"=FALSE ("R6 (B/DIO13 (Pin 26))"), "J4 UP"=FALSE ("R5 (B/DIO4 (Pin 19))"), "J3 DOWN"=FALSE ("R4 (B/DIO3 (Pin 17))"), "J3 UP"=FALSE ("R7 (B/DIO14 (Pin 32))"), "J2 DOWN"=FALSE ("R8 (B/DIO15 (Pin 34))"), "J2 UP"=FALSE ("R1 (B/DIO0 (Pin 11))"), "J1 DOWN"=FALSE ("R2 (B/DIO1 (Pin 13))"), "J1 UP"=FALSE ("R3 (B/DIO2 (Pin 15))")) -> ()
                          }
                        }
                      }
                    }
                    n242 = Increment(x=w507) -> (x+1=w506:i32)
                  }
                }
              }
            }
          }
        }
      }
      frame #2 {
        n243 = local read "Temp"() -> (w822:dbl)
        n244 = Wait (ms)(milliseconds to wait=u32 10) -> ()  [unwired: 1 out]
        n245 = Not Equal?(x=w822, y=0.0) -> (x != y?=w821:bool)
        n246 = case shown="True" w821 {
          frame False {
          }
          frame True {
            n247 = local read "X Axis"() -> (w827:dbl)
            n248 = Multiply(x=w827, y=10.0) -> (x*y=w825:dbl)
            n249 = To Word Integer(number=w825) -> (16bit integer=w824:i16)
            n250 = Format Into String(initial string="x0.val=", w824) -> (resulting string=w828:string)  [unwired: 2 in, 1 out]
            n251 = call "Nextion_Write.vi"("string"=w828) -> ()  [unwired: 10 in, 1 out]
          }
        }
      }
      frame #3 {
        n252 = local read "Temp"() -> (w833:dbl)
        n253 = Wait (ms)(milliseconds to wait=u32 10) -> ()  [unwired: 1 out]
        n254 = Not Equal?(x=w833, y=0.0) -> (x != y?=w834:bool)
        n255 = case shown="True" w834 {
          frame False {
          }
          frame True {
            n256 = local read "Y Axis"() -> (w839:dbl)
            n257 = Multiply(x=w839, y=10.0) -> (x*y=w837:dbl)
            n258 = To Word Integer(number=w837) -> (16bit integer=w836:i16)
            n259 = Format Into String(initial string="x1.val=", w836) -> (resulting string=w840:string)  [unwired: 2 in, 1 out]
            n260 = call "Nextion_Write.vi"("string"=w840) -> ()  [unwired: 10 in, 1 out]
          }
        }
      }
      frame #4 {
        # "Generate warning for deviation in level"
        n261 = local read "levell check"() -> (w848:i32)
        n262 = call "Nextion_PageRead.vi"() -> ("pageNo"=w844:u8)  [unwired: 10 in, 1 out]
        n263 = Equal?(x=w844, y=u8 0) -> (x = y?=w842:bool)
        n264 = Equal?(x=w848, y=1) -> (x = y?=w845:bool)
        n265 = And(x=w842, y=w845) -> (x .and. y?=w846:bool)
        n266 = case shown="False" w846 {
          frame False {
            n267 = Format Into String(initial string="t2.bco=", 65535 ("input 1")) -> (resulting string=w853:string)  [unwired: 2 in, 1 out]
            n268 = call "Nextion_Write.vi"("string"=w853) -> ()  [unwired: 10 in, 1 out]
          }
          frame True {
            n269 = local read "X Axis"() -> (w858:dbl)
            n270 = local read "Y Axis"() -> (w859:dbl)
            n271 = local read "Temp"() -> (w860:dbl)
            n272 = Not Equal To 0?(x=w860) -> (x != 0?=w854:bool)
            n273 = call "Truck_inclination_quadrantFind.vi"("y"=w859, "x"=w858) -> ("z"=w857:i16)  [unwired: 9 in]
            n274 = Not Equal To 0?(x=w857) -> (x != 0?=w855:bool)
            n275 = And(x=w854, y=w855) -> (x .and. y?=w856:bool)
            n276 = case shown="True" w856 {
              frame False {
              }
              frame True {
                n277 = Format Into String(initial string="t2.bco=", 32768 ("input 1")) -> (resulting string=w863:string)  [unwired: 2 in, 1 out]
                n278 = call "Nextion_Write.vi"("string"=w863) -> ()  [unwired: 10 in, 1 out]
              }
            }
          }
        }
      }
    }
    "Numeric" <- w15
  }
  n279 = while {
    i -> [w868]
    stop <- FALSE ("stop 2") stop-if-true
    n280 = xnode "MANUAL/SFTWRE"() -> ("MANUAL/SFTWRE SELECT (B/DIO8 (Pin 27))"=w864:bool)  [unwired: 1 in, 1 out]
    n281 = Wait (ms)(milliseconds to wait=u32 100) -> ()  [unwired: 1 out]
    n282 = Not(x=w864) -> (.not. x?=w865:bool)
    n283 = case shown="False" w865 {
      frame False {
        n284 = flat-sequence {
          frame #0 {
            n285 = Wait (ms)(milliseconds to wait=u32 50) -> ()  [unwired: 1 out]
            n286 = call "motor_ctrl.vi"("Motor"=FALSE ("contactor (A/DIO3 (Pin 17))")) -> ()  [unwired: 7 in]
          }
          frame #1 {
            n287 = Wait (ms)(milliseconds to wait=u32 50) -> ()  [unwired: 1 out]
            n288 = call "interlock_ctrl.vi"("Interlock"=FALSE ("interlock_relay (B/DIO8 (Pin 27))")) -> ()  [unwired: 7 in]
          }
          frame #2 {
            n289 = call "jacks_out_v3.vi"("J4 DOWN"=FALSE ("R6 (B/DIO13 (Pin 26))"), "J4 UP"=FALSE ("R5 (B/DIO4 (Pin 19))"), "J3 DOWN"=FALSE ("R4 (B/DIO3 (Pin 17))"), "J3 UP"=FALSE ("R7 (B/DIO14 (Pin 32))"), "J2 DOWN"=FALSE ("R8 (B/DIO15 (Pin 34))"), "J2 UP"=FALSE ("R1 (B/DIO0 (Pin 11))"), "J1 DOWN"=FALSE ("R2 (B/DIO1 (Pin 13))"), "J1 UP"=FALSE ("R3 (B/DIO2 (Pin 15))")) -> ()
          }
        }
      }
      frame True {
        n290 = call "interlock_ctrl.vi"("Interlock"=TRUE ("interlock_relay (B/DIO8 (Pin 27))")) -> ()  [unwired: 7 in]
      }
    }
    "Numeric 2" <- w868
  }
  n291 = disable-structure shown="Disabled" {
    frame Disabled {
      n292 = while {
        stop <- FALSE ("stop 3") stop-if-true
        n293 = call "InclinometerMeter.vi"() -> ("Temp"=→"Temp":dbl, "Y Axis"=w934:dbl, "X Axis"=w933:dbl)  [unwired: 9 in]
        n294 = Wait (ms)(milliseconds to wait=u32 200) -> ()  [unwired: 1 out]
        n295 = Negate(x=w934) -> (-x=w931:dbl)
        n296 = Subtract(x=w933, y=0.3) -> (x-y=w923:dbl)
        n297 = Subtract(x=w931, y=-1.3) -> (x-y=w917:dbl)
        n298 = Less Or Equal?(x=w923, y=0.3) -> (x <= y?=w925:bool)
        n299 = Less Or Equal?(x=w917, y=0.2) -> (x <= y?=w920:bool)
        n300 = Select(t=0.0, s=w925, f=w923) -> (s? t:f=→"X Axis":dbl)
        n301 = Select(t=0.0, s=w920, f=w917) -> (s? t:f=→"Y Axis":dbl)
      }
    }
    frame Enabled {
    }
  }
